vi "DefPapeis.vi"(6 "IA State Output":T2 {"enemy_robots"."Agentes Disponíveis" format="%#_13g"; "our_robots"."Agentes Disponíveis" format="%#_13g"}, 7 "InfoMissao":T13 {"Agentes Disponíveis" format="%#_13g"}, 10 "Boolean":bool, 11 "channel":T14) -> (2 "channel info":T1, 3 "channel 2":T14)   [LabVIEW 2018]
uses:
  <extravilib>/ChannelInstances/Lossy Stream-t'AI Input.ctl'/)Channel.ctl
  Core/AI Input.ctl
  Core/AI Robot.ctl
  Intel/Functions Enum.ctl
  Intel/AttackerStates.ctl
  Path Planning/RRT/PathDests.ctl
  Path Planning/RRT/PathDest.ctl
  Core/AI Ball.ctl
  Core/Field Size.ctl
  Core/AI Judge.ctl
  Intel/Command Enum.ctl
  Util/Events/Events.ctl
  InfoMissao.ctl
  <extravilib>/ChannelInstances/Lossy Stream-t'InfoMissao.ctl'/)Channel.ctl
  <extravilib>/ChannelInstances/Lossy Stream-t'InfoMissao.ctl'/Write With Abort.vi
  <extravilib>/ChannelInstances/Lossy Stream-t'AI Input.ctl'/Read With Abort.vi
  <extravilib>/ChannelInstances/Lossy Stream-t'AI Input.ctl'/Write With Abort.vi
  <extravilib>/ChannelInstances/Lossy Stream-t'InfoMissao.ctl'/Endpoint.vi
  <extravilib>/ChannelInstances/Lossy Stream-t'AI Input.ctl'/EndpointRead.vi
  <extravilib>/ChannelInstances/Lossy Stream-t'AI Input.ctl'/Endpoint.vi
  <extravilib>/ChannelInstances/Lossy Stream-t'AI Input.ctl'/)Channel.vi
  <resource>/ChannelSupport/_ChannelSupport/WaitIfNeeded.vi
  <extravilib>/ChannelInstances/Lossy Stream-t'InfoMissao.ctl'/)Channel.vi
  <extravilib>/ChannelInstances/Lossy Stream-t'AI Input.ctl'.lvlib
  <extravilib>/ChannelInstances/Lossy Stream-t'InfoMissao.ctl'.lvlib
panel:
  out "Output IA":T2 {"enemy_robots"."Agentes Disponíveis" format="%#_13g"; "our_robots"."Agentes Disponíveis" format="%#_13g"}
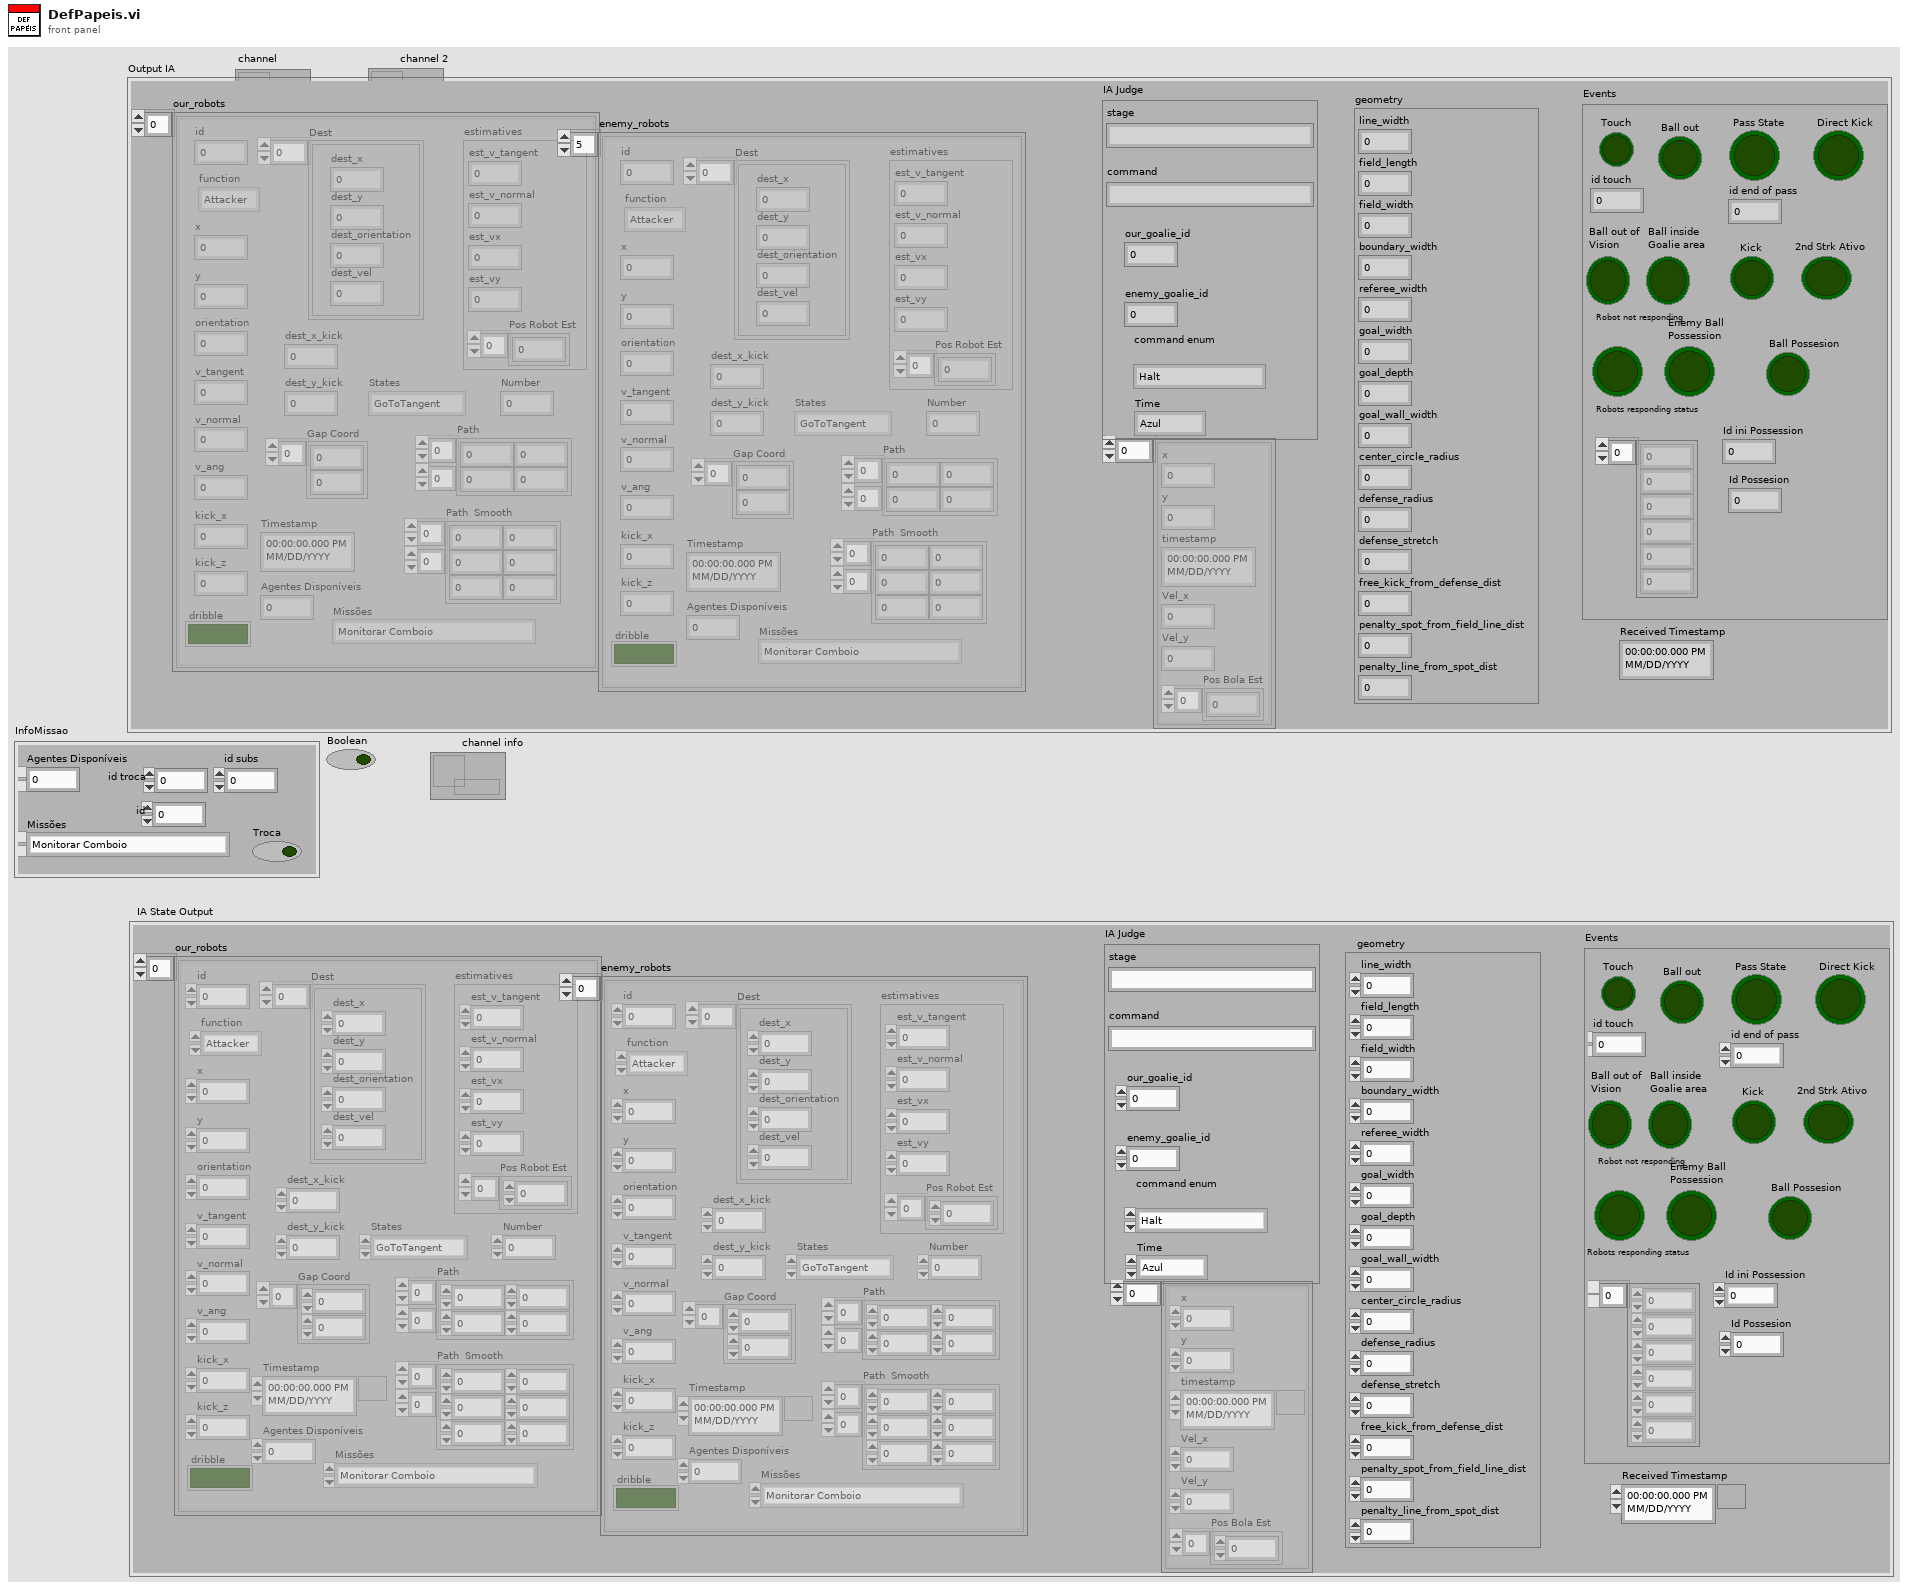
[diagram p1: front panel]
types:
  T1 = typedef "Lossy Stream-t'InfoMissao.ctl'.lvlib/)Channel.ctl" = refnum<queue>
  T2 = typedef "AI Input.ctl" = cluster{"our_robots":T3[], "enemy_robots":T3[], "balls":T8[], "geometry":T9, "IA Judge":T10, "Received Timestamp":timestamp, "Events":T12}
  T3 = typedef "AI Robot.ctl" = cluster{"id":u32, "function":T4, "x":dbl, "y":dbl, "orientation":dbl, "v_tangent":dbl, "v_normal":dbl, "v_ang":dbl, "kick_x":dbl, "kick_z":dbl, "dribble":bool, "Timestamp":timestamp, "estimatives":cluster{"est_v_tangent":dbl, "est_v_normal":dbl, "est_vx":dbl, "est_vy":dbl, "Pos Robot Est":dbl[]}, "dest_x_kick":dbl, "dest_y_kick":dbl, "Gap Coord":dbl[], "States":T5, "Path ":dbl[][], "Path  Smooth":dbl[][], "Dest":T6, "Missões ":enum16{"Monitorar Comboio", "Realizar Segurança de Retaguarda", "Vigiar Área", "Reconhecimento de Área"}, "Agentes Disponíveis":dbl, "Number":dbl}
  T4 = typedef "Functions Enum.ctl" = enum16{"None", "Vigia", "2nd Striker", "Attacker", "Goalie", "Defender", "Striker", "Goto 0", "Dummy", "Kicker", "ZigZag 0", "ZigZag 1", "ZigZag 2", "ZigZag 3", "ZigZag 4", "ZigZag 5", "ZigZag 6", "ZigZag 7", "ZigZag 8", ""}
  T5 = typedef "AttackerStates.ctl" = enum16{"Pass", "GoToTangent", "BallGetting", "GoToKick", ""}
  T6 = typedef "PathDests.ctl" = T7[]
  T7 = typedef "PathDest.ctl" = cluster{"dest_x":dbl, "dest_y":dbl, "dest_orientation":dbl, "dest_vel":dbl}
  T8 = typedef "AI Ball.ctl" = cluster{"x":dbl, "y":dbl, "timestamp":timestamp, "Vel_x":dbl, "Vel_y":dbl, "Pos Bola Est":dbl[]}
  T9 = typedef "Field Size.ctl" = cluster{"line_width":u32, "field_length":u32, "field_width":u32, "boundary_width":u32, "referee_width":u32, "goal_width":u32, "goal_depth":u32, "goal_wall_width":u32, "center_circle_radius":u32, "defense_radius":u32, "defense_stretch":u32, "free_kick_from_defense_dist":u32, "penalty_spot_from_field_line_dist":u32, "penalty_line_from_spot_dist":u32}
  T10 = typedef "AI Judge.ctl" = cluster{"stage":string, "command":string, "our_goalie_id":dbl, "enemy_goalie_id":dbl, "command enum":T11, "Time":enum16{"Azul", "Amarelo"}}
  T11 = typedef "Command Enum.ctl" = enum16{"Halt", "Stop", "Force Start", "PKA Normal Start", "Prepare Kickoff Ally", "PKE Normal Start", "Prepare Kickoff Enemy", "Prepare Penalty Ally", "PPA Normal Start", "Prepare Penalty Enemy", "PPE Normal Start", "Direct Free Enemy", "Direct Free Ally", "Indirect Free Enemy", "Indirect Free Ally", "Timeout Enemy", "Timeout Ally", "Goal Enemy", "Goal Ally", "Ball Placement Enemy", "Ball Placement Ally", "Normal Half Time", "Extra Time Break", "Extra Half Time", "None", "Post Game"}
  T12 = typedef "Events.ctl" = cluster{"Touch":bool, "Ball out":bool, "id touch":dbl, "Ball out of \nVision":bool, "Ball inside \nGoalie area":bool, "Robot not responding":bool, "Robots responding status":dbl[], "Enemy Ball \nPossession":bool, "Pass State":bool, "id end of pass":dbl, "Kick":bool, "Id ini Possession":dbl, "Ball Possesion":bool, "Id Possesion":dbl, "Direct Kick":bool, "2nd Strk Ativo":bool}
  T13 = typedef "InfoMissao.ctl" = cluster{"Troca ":bool, "Missões ":enum16{"Monitorar Comboio", "Realizar Segurança de Retaguarda", "Vigiar Área", "Reconhecimento de Área"}, "Agentes Disponíveis":dbl, "id troca ":dbl, "id subs":dbl, "id ":dbl}
  T14 = typedef "Lossy Stream-t'AI Input.ctl'.lvlib/)Channel.ctl" = refnum<queue>
  T15 = enum16{"Monitorar Comboio", "Realizar Segurança de Retaguarda", "Vigiar Área", "Reconhecimento de Área"}
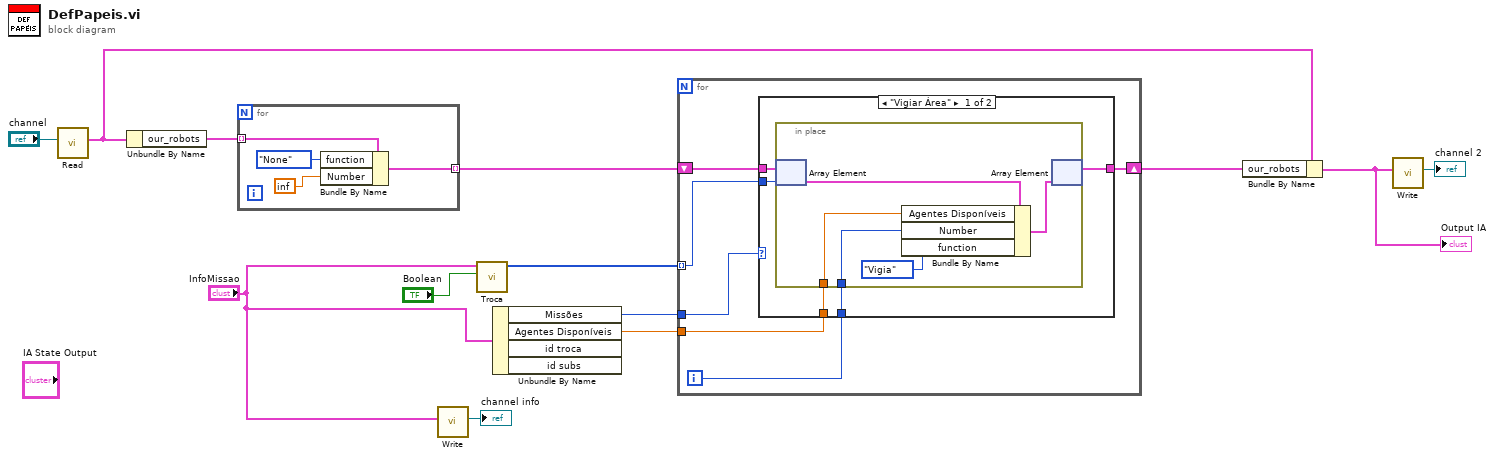
[diagram p0: block diagram]
diagram:
  n1 = call <extravilib>:"Read.vi"("channel"="channel") -> ("element"=w5:T2)  [unwired: 5 in, 5 out]
  n2 = Unbundle By Name(w5) -> ("our_robots"=w11:T3[])
  n3 = for {
    tunnel: w11 -> [w17] mode=indexing
    tunnel: [w16] -> w9 mode=indexing
    n4 = Bundle By Name(cluster=w17, "function"=Functions_Enum."None", "Number"=inf) -> (w16:T3)
  }
  n5 = call <extravilib>:"Write.vi"("element"="InfoMissao") -> ("channel"=→"channel info":T1)  [unwired: 8 in, 2 out]
  n6 = call "Troca.vi"("first call"="Boolean", "InfoMissao"="InfoMissao") -> ("Vetor de Agentes"=w8:i32[])  [unwired: 9 in]
  n7 = Unbundle By Name("InfoMissao") -> ("Missões"=w6:T15, "Agentes Disponíveis"=w7:dbl)  [unwired: 2 out]
  n8 = for {
    tunnel: w8 -> [w22] mode=indexing
    tunnel: w7 -> [w21]
    tunnel: w6 -> [w19]
    shift-right: [w18] -> w4
    shift-left: w9 -> [w23]
    i -> [w20]
    n9 = case shown="\"Vigiar Área\"" w19 {
      tunnel: w23 -> [w28 w34]
      tunnel: w22 -> [w27 _]
      tunnel: w21 -> [w26 _]
      tunnel: w20 -> [w25 _]
      tunnel: [w24 w34] -> w18
      frame "Vigiar Área" {
        n10 = in-place {
          in-place-border: w26 -> [w31]
          in-place-border: w25 -> [w30]
          n11 = in-place-array #1(w28, w27) -> (w33:T3)
          n12 = Bundle By Name(cluster=w33, "Agentes Disponíveis"=w31, "Number"=w30, "function"=Functions_Enum."Vigia") -> (w32:T3)
          n13 = in-place-array #1(w32) -> (w24:T3[])  [unwired: 1 out]
        }
      }
      frame Default {
      }
    }
  }
  n14 = Bundle By Name(cluster=w5, "our_robots"=w4) -> (w3:T2)
  "Output IA" <- w3
  n15 = call <extravilib>:"Write.vi"("element"=w3) -> ("channel"=→"channel 2":T14)  [unwired: 8 in, 2 out]
